vi "Joystick adjustments.vi"(10 "Speed":dbl, 11 "Turn":dbl) -> (2 "Right Motor Value":dbl, 3 "Left Motor Value":dbl)   [LabVIEW 2017]
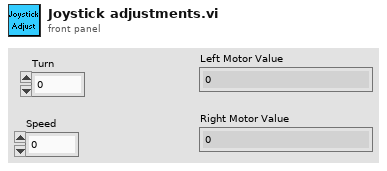
[diagram p1: front panel]
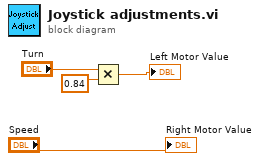
[diagram p0: block diagram]
diagram:
  n1 = Multiply(x="Turn", y=0.84) -> (x*y=→"Left Motor Value":dbl)
  "Right Motor Value" <- "Speed"
